vi "Bezier Trajectory.vi"(6 "Overrides":T1 {"Angle Override" step=5.0; "Velocity Override" step=5.0; "Angular Override" step=5.0}, 7 "Drive Type":T4, 8 "Conditions":T7, 9 "All Limits":cluster{"Limits":T2, "Angular Limits":T3} {"Limits"."StoopidFast (fps)" min=0.0; "Limits"."Jerk (fps^3)" min=0.0 step=1.0; "Limits"."Accel (fps^2)" min=0.0; "Limits"."Velocity (fps)" min=0.0; "Angular Limits"."Jerk (deg/s^3)" min=0.0 step=1.0; "Angular Limits"."Accel (deg/s^2)" min=0.0; "Angular Limits"."Velocity (deg/s)" min=0.0}, 10 "sample period (s)":sgl, 11 "WayPoints":T8) -> (0 "Time & Dist":cluster{"Time (s)":dbl, "Distance (ft)":dbl}, 1 "Valid":bool, 2 "Updated Waypoints":cluster{"x":dbl, "y":dbl, "th":dbl}[](array[cluster]), 3 "Trajectory Data":T5)   [LabVIEW 2023]
uses:
  Types/Waypoints.ctl
  Types/Trajectory Data.ctl
  Types/Segment Type.ctl
  Types/Drive Type.ctl
  Types/Limits.ctl
  Types/Angluar Limits.ctl
  Types/Overrides.ctl
panel:
  out "XY Graph":cluster{"X":dbl, "Y":dbl}[](graph)
  in  "dynamic?":bool
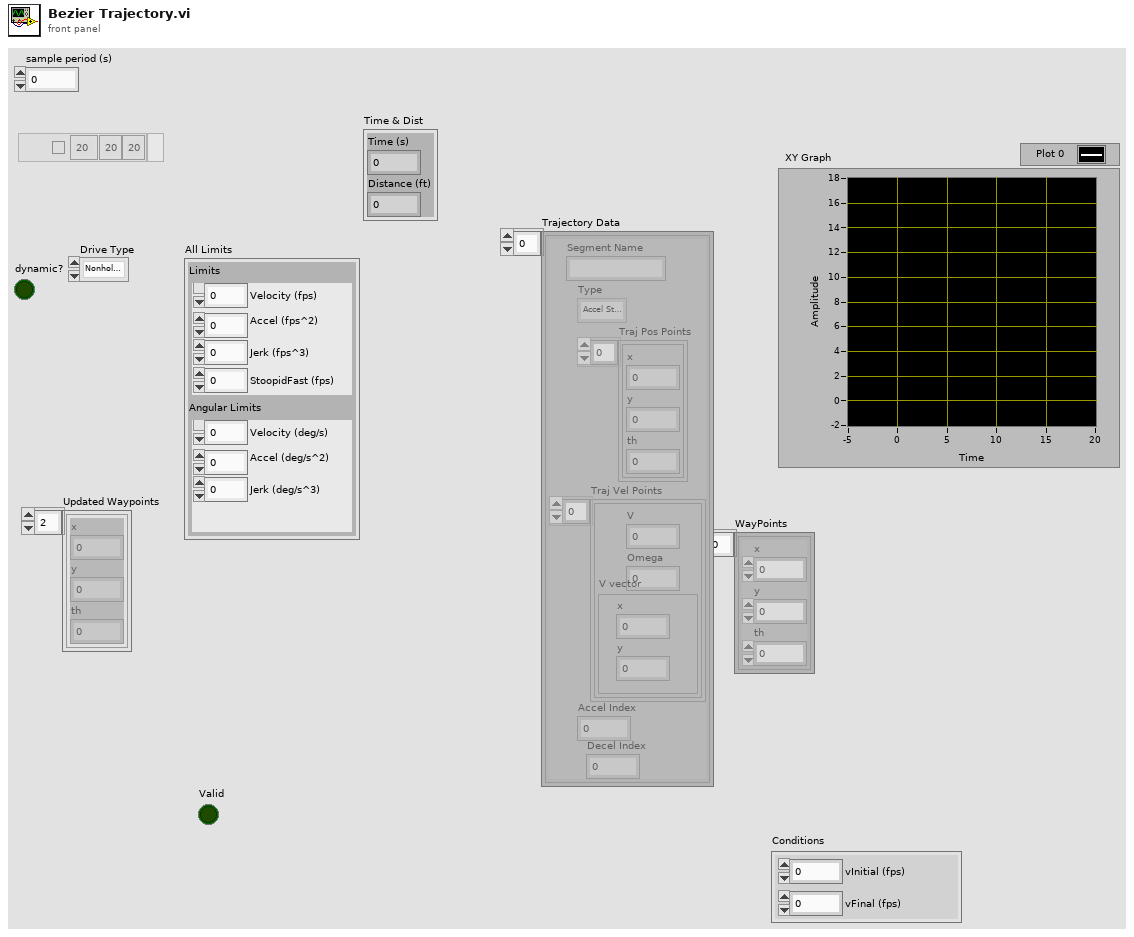
[diagram p1: front panel]
types:
  T1 = typedef "Overrides.ctl" = cluster{"Count":string, "Angular Override":dbl, "Enabled?":bool, "Velocity Override":dbl, "Angle Override":dbl}[]
  T2 = typedef "Limits.ctl" = cluster{"Velocity (fps)":dbl, "Accel (fps^2)":dbl, "Jerk (fps^3)":dbl, "StoopidFast (fps)":dbl}
  T3 = typedef "Angluar Limits.ctl" = cluster{"Velocity (deg/s)":dbl, "Accel (deg/s^2)":dbl, "Jerk (deg/s^3)":dbl}
  T4 = typedef "Drive Type.ctl" = enum16{"Nonholonomic", "Holonomic"}
  T5 = typedef "Trajectory Data.ctl" = cluster{"Segment Name":string, "Type":T6, "Traj Pos Points":cluster{"x":dbl, "y":dbl, "th":dbl}[], "Traj Vel Points":cluster{"V":dbl, "Omega":dbl, "V vector":cluster{"y":dbl, "x":dbl}}[], "Accel Index":i32, "Decel Index":i32}[]
  T6 = typedef "Segment Type.ctl" = enum16{"Accel Straight", "Const Straight", "Blend", "Circle", "Bezier"}
  T7 = cluster{"vInitial (fps)":dbl, "vFinal (fps)":dbl}
  T8 = typedef "Waypoints.ctl" = cluster{"x":sgl, "y":sgl, "th":sgl}[]
  T9 = cluster{"Velocity (fps)":dbl, "Accel (fps^2)":dbl, "Jerk (fps^3)":dbl}
  T10 = typedef "Bezier Curve.ctl" = cluster{"x":sgl, "y":sgl}[]
  T11 = cluster{"Segment Name":string, "Type":T6, "Traj Pos Points":cluster{"x":dbl, "y":dbl, "th":dbl}[], "Traj Vel Points":cluster{"V":dbl, "Omega":dbl, "V vector":cluster{"y":dbl, "x":dbl}}[], "Accel Index":i32, "Decel Index":i32}
  T12 = cluster{"Segment Name":string, "Type":T6, "Traj Pos Points":cluster{"x":dbl, "y":dbl, "th":dbl}[], "Traj Vel Points":cluster{"V":dbl, "Omega":dbl, "V vector":cluster{"y":dbl, "x":dbl}}[], "Accel Index":i32, "Decel Index":i32}[]
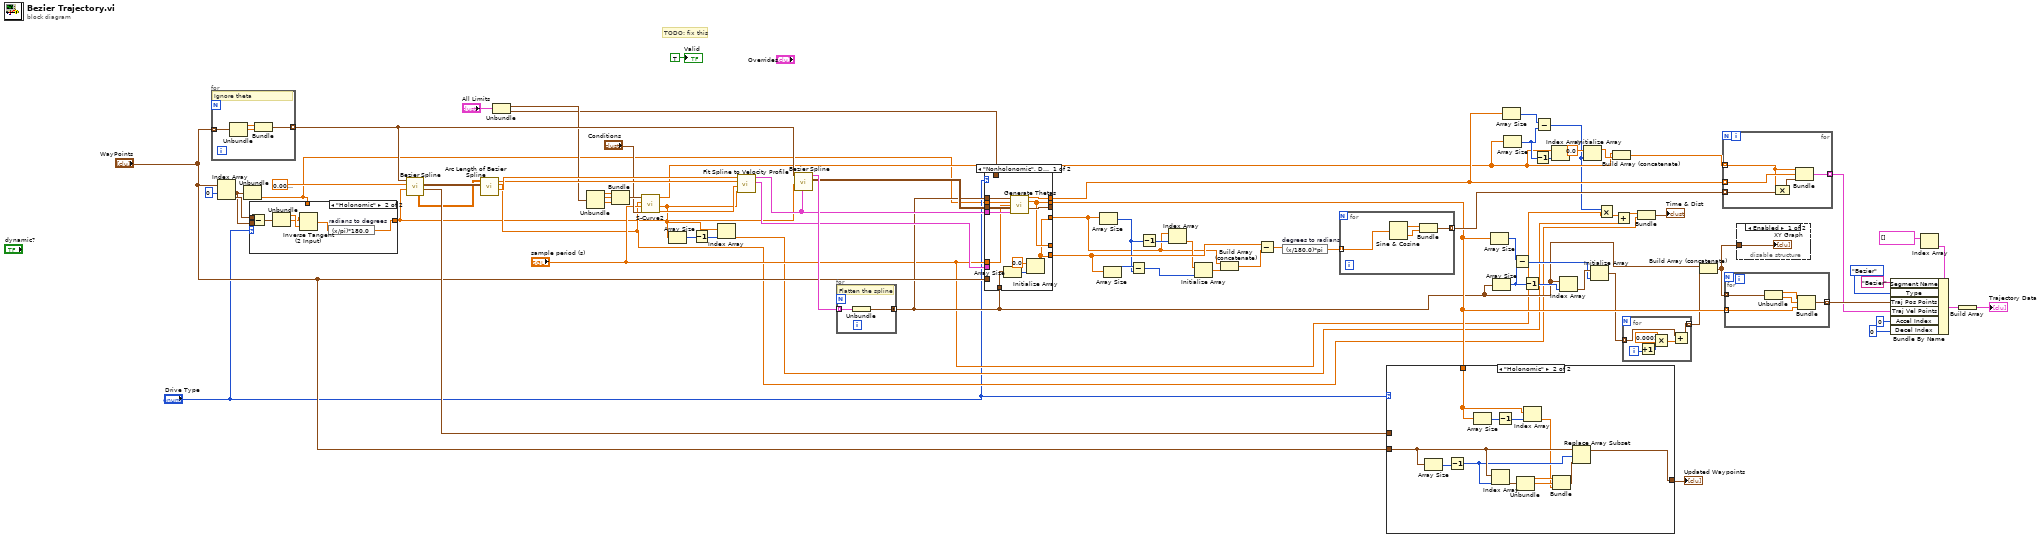
[diagram p0: block diagram]
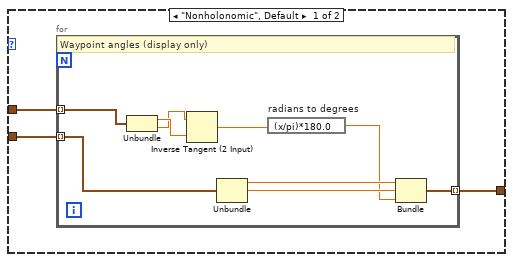
[diagram p4: hidden frame]
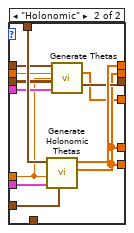
[diagram p5: hidden frame]
diagram:
  # "TODO: fix this"
  n1 = for {
    tunnel: "WayPoints" -> [w83] mode=indexing
    tunnel: [w80] -> w61 mode=indexing
    # "Ignore theta"
    n2 = Unbundle(w83) -> ("x"=w82:sgl, "y"=w81:sgl)  [unwired: 1 out]
    n3 = Bundle("x"=w82, "y"=w81) -> (w80:cluster{"x":sgl, "y":sgl})  [unwired: 1 in]
  }
  n4 = Index Array(array="WayPoints", index #1=0 ("index")) -> (element #1=w4:cluster{"x":sgl, "y":sgl, "th":sgl}, element #2=w5:cluster{"x":sgl, "y":sgl, "th":sgl})  [unwired: 1 in]
  n5 = Unbundle(w4) -> ("th"=w2:sgl)  [unwired: 2 out]
  n6 = case shown="\"Holonomic\"" "Drive Type" {
    tunnel: w5 -> [_ w91]
    tunnel: w4 -> [_ w90]
    tunnel: [w84 w85] -> w1
    tunnel: w2 -> [w84 _]
    frame "Nonholonomic", Default {
    }
    frame "Holonomic" {
      n7 = Subtract(x=w91, y=w90) -> (x-y=w89:cluster{"x":sgl, "y":sgl, "th":sgl})
      n8 = Unbundle(w89) -> ("x"=w88:sgl, "y"=w87:sgl)  [unwired: 1 out]
      n9 = Inverse Tangent (2 Input)(1:w88, 2:w87) -> (0:w86:sgl)
      n10 = expression code="(x/pi)*180.0" "radians to degrees"(w86) -> (w85:sgl)
    }
  }
  n11 = call "Bezier Spline.vi"("starting orientation (deg)"=w1, "percision"=sgl 0.01, "waypts"=w61) -> ("Tangents"=w74:cluster{sgl, sgl}[], "ctrl pts"=w64:cluster{sgl, sgl}[][], "position out"=w58:sgl[][])  [unwired: 4 in, 2 out]
  n12 = call "Arc Length of Bezier Spline.vi"("ctrl pts"=w64, "position"=w58) -> ("t"=w63:sgl[], "l total"=w8:dbl, "l"=w62:dbl[])  [unwired: 6 in, 1 out]
  n13 = Unbundle("All Limits") -> ("Limits"=w51:T2, "Angular Limits"=w50:T3)
  n14 = Unbundle(w51) -> ("Velocity (fps)"=w78:dbl, "Accel (fps^2)"=w77:dbl, "Jerk (fps^3)"=w76:dbl)  [unwired: 1 out]
  n15 = Bundle("Velocity (fps)"=w78, "Accel (fps^2)"=w77, "Jerk (fps^3)"=w76) -> (w75:T9)  [unwired: 1 in]
  n16 = call "S-Curve2.vi"("Conditions"="Conditions", "dt (s)"="sample period (s)", "goal"=w8, "Limits"=w75) -> ("X"=w60:dbl[], "T"=w54:dbl[], "V"=w18:dbl[])  [unwired: 5 in]
  n17 = Array Size(array=w54) -> (size(s)=w73:i32)
  n18 = Decrement(x=w73) -> (x-1=w72:i32)
  n19 = Index Array(array=w54, index=w72) -> (element=w9:dbl)
  n20 = call "Fit Spline to Velocity Profile.vi"("time"=w54, "vel positions"=w60, "s(t)"=w62, "t flat"=w63) -> ("time unflat"=w53:cluster{dbl[]}[], "y unflat"=w55:cluster{dbl[]}[])  [unwired: 6 in]
  n21 = call "Bezier Spline.vi"("positions"=w55, "starting orientation (deg)"=w1, "waypts"=w61) -> ("ctrl pts"=w56:cluster{sgl, sgl}[][], "bezier spline"=w57:cluster{"curve ":T10}[])  [unwired: 4 in, 3 out]
  n22 = for {
    tunnel: w57 -> [w93] mode=indexing
    tunnel: [w92] -> w34 mode=concatenating
    # "Flatten the spline"
    n23 = Unbundle(w93) -> ("curve"=w92:T10)
  }
  n24 = case shown="\"Nonholonomic\", Default" "Drive Type" {
    tunnel: [w105 w117] -> w24
    tunnel: [w99 w108] -> w40
    tunnel: w2 -> [w104 w112]
    tunnel: w34 -> [w103 w113]
    tunnel: w56 -> [w102 w111]
    tunnel: w55 -> [w101 w110]
    tunnel: w53 -> [_ w116]
    tunnel: "sample period (s)" -> [w94 w106]
    tunnel: w50 -> [_ w115]
    tunnel: "WayPoints" -> [_ w114]
    tunnel: [w100 w109] -> _
    tunnel: [w99 w108] -> _
    tunnel: [w95 w108] -> w33
    tunnel: [w95 w107] -> w27
    tunnel: w34 -> [w98 _]
    frame "Nonholonomic", Default {
      n25 = Array Size(array=w98) -> (size(s)=w97:i32)
      n26 = call "Generate Thetas.vi"("spline flat"=w103, "starting angle"=w104, "dt"=w94, "ctrl pts"=w102, "y unflat"=w101) -> ("omega"=w105:sgl[], "theta"=w99:sgl[], "Tangent Vector"=w100:cluster{"x out":dbl, "y out":dbl}[])  [unwired: 8 in]
      n27 = Initialize Array(0.0 ("element"), w97) -> (w95:dbl[])
    }
    frame "Holonomic" {
      n28 = call "Generate Holonomic Thetas.vi"("WayPoints"=w114, "time unflat"=w116, "dt"=w106, "Angular Limits"=w115) -> ("X"=w108:dbl[], "V"=w117:dbl[])  [unwired: 6 in]
      n29 = call "Generate Thetas.vi"("spline flat"=w113, "starting angle"=w112, "dt"=w106, "ctrl pts"=w111, "y unflat"=w110) -> ("theta"=w107:sgl[], "Tangent Vector"=w109:cluster{"x out":dbl, "y out":dbl}[])  [unwired: 8 in, 1 out]
    }
  }
  n30 = Array Size(array=w27) -> (size(s)=w30:i32)
  n31 = Array Size(array=w33) -> (size(s)=w32:i32)
  n32 = Subtract(x=w32, y=w30) -> (x-y=w31:i32)
  n33 = Decrement(x=w30) -> (x-1=w29:i32)
  n34 = Index Array(array=w27, index=w29) -> (element=w28:dbl)
  n35 = Initialize Array(w28, w31) -> (w26:dbl[])
  n36 = Build Array (concatenate)(w27, w26) -> (w25:dbl[])
  n37 = Subtract(x=w33, y=w25) -> (x-y=w41:dbl[])
  n38 = expression code="(x/180.0)*pi" "degrees to radians"(w41) -> (w42:dbl[])
  n39 = for {
    tunnel: w42 -> [w119] mode=indexing
    tunnel: [w121] -> w43 mode=indexing
    n40 = Sine & Cosine(0:w119) -> (1:w120:dbl, 2:w118:dbl)
    n41 = Bundle(w120, w118) -> (w121:cluster{dbl, dbl})  [unwired: 1 in]
  }
  n42 = case shown="\"Holonomic\"" "Drive Type" {
    tunnel: w74 -> [w124 _]
    tunnel: "WayPoints" -> [w123 w141]
    tunnel: [w122 w134] -> w49
    tunnel: w40 -> [_ w143]
    frame "Nonholonomic", Default {
      n43 = for {
        tunnel: w123 -> [w133] mode=indexing
        tunnel: w124 -> [w125] mode=indexing
        tunnel: [w130] -> w122 mode=indexing
        # "Waypoint angles (display only)"
        n44 = Unbundle(w125) -> (w128:sgl, w127:sgl)
        n45 = Inverse Tangent (2 Input)(1:w128, 2:w127) -> (0:w126:sgl)
        n46 = Unbundle(w133) -> ("x"=w132:sgl, "y"=w131:sgl)  [unwired: 1 out]
        n47 = expression code="(x/pi)*180.0" "radians to degrees"(w126) -> (w129:sgl)
        n48 = Bundle("x"=w132, "y"=w131, w129) -> (w130:cluster{"x":sgl, "y":sgl, sgl})  [unwired: 1 in]
      }
    }
    frame "Holonomic" {
      n49 = Array Size(array=w141) -> (size(s)=w142:i32)
      n50 = Decrement(x=w142) -> (x-1=w140:i32)
      n51 = Array Size(array=w143) -> (size(s)=w145:i32)
      n52 = Index Array(array=w141, index=w140) -> (element=w139:cluster{"x":sgl, "y":sgl, "th":sgl})
      n53 = Decrement(x=w145) -> (x-1=w144:i32)
      n54 = Unbundle(w139) -> ("x"=w138:sgl, "y"=w137:sgl)  [unwired: 1 out]
      n55 = Index Array(array=w143, index=w144) -> (element=w136:dbl)
      n56 = Bundle("x"=w138, "y"=w137, w136) -> (w135:cluster{"x":sgl, "y":sgl, dbl})  [unwired: 1 in]
      n57 = Replace Array Subset(array=w141, new element=w135, index=w140) -> (w134:T8)
    }
  }
  "Updated Waypoints" <- w49
  n58 = Array Size(array=w40) -> (size(s)=w39:i32)
  n59 = Array Size(array=w34) -> (size(s)=w38:i32)
  n60 = Array Size(array=w24) -> (size(s)=w23:i32)
  n61 = Array Size(array=w18) -> (size(s)=w22:i32)
  n62 = Subtract(x=w39, y=w38) -> (x-y=w35:i32)
  n63 = Decrement(x=w38) -> (x-1=w37:i32)
  n64 = Decrement(x=w22) -> (x-1=w21:i32)
  n65 = Subtract(x=w23, y=w22) -> (x-y=w14:i32)
  n66 = Index Array(array=w18, index=w21) -> ()  [unwired: 1 out]
  n67 = Index Array(array=w34, index=w37) -> (element=w36:cluster{"x":sgl, "y":sgl})
  n68 = Initialize Array(0.0 ("element"), w14) -> (w20:dbl[])
  n69 = Initialize Array(w36, w35) -> (w16:cluster{"x":sgl, "y":sgl}[])
  n70 = Multiply(x=w14, y="sample period (s)") -> (x*y=w13:sgl)
  n71 = Build Array (concatenate)(w18, w20) -> (w17:dbl[])
  n72 = Add(x=w13, y=w9) -> (x+y=w12:dbl)
  n73 = for {
    tunnel: w16 -> [w147] mode=indexing
    tunnel: [w146] -> w15 mode=indexing
    i -> [w150]
    n74 = Increment(x=w150) -> (x+1=w149:i32)
    n75 = Multiply(x=0.0001, y=w149) -> (x*y=w148:dbl)
    n76 = Add(x=w147, y=w148) -> (x+y=w146:cluster{"x":dbl, "y":dbl})
  }
  n77 = Bundle(w12, "l total"=w8) -> (→"Time & Dist":cluster{dbl, "l total":dbl})  [unwired: 1 in]
  n78 = Build Array (concatenate)(w34, w15) -> (w7:cluster{"x":dbl, "y":dbl}[])
  n79 = for {
    tunnel: w24 -> [w156] mode=indexing
    tunnel: w17 -> [w152] mode=indexing
    tunnel: [w155] -> w67 mode=indexing
    tunnel: w43 -> [w153] mode=indexing
    n80 = Compound Arithmetic op=MULTIPLY(w152, w153) -> (w154:cluster{dbl, dbl})
    n81 = Bundle("element"=w152, w156, w154) -> (w155:cluster{"element":dbl, dbl, cluster{dbl, dbl}})  [unwired: 1 in]
  }
  n82 = for {
    tunnel: w7 -> [w161] mode=indexing
    tunnel: [w158] -> w68 mode=indexing
    tunnel: w40 -> [w157] mode=indexing
    n83 = Unbundle(w161) -> ("x"=w160:dbl, "y"=w159:dbl)
    n84 = Bundle("x"=w160, "y"=w159, w157) -> (w158:cluster{"x":dbl, "y":dbl, dbl})  [unwired: 1 in]
  }
  n85 = disable-structure shown="Enabled" {
    disable-tunnel: w7 -> [w162 _]
    frame Enabled {
      "XY Graph" <- w162
    }
    frame Disabled {
    }
  }
  n86 = Index Array(array=T5 [] ("Trajectory Data")) -> (element=w44:T11)  [unwired: 1 in]
  n87 = Bundle By Name(cluster=w44, "Segment Name"="Bezier", "Type"=Segment_Type."Bezier", "Traj Pos Points"=w68, "Traj Vel Points"=w67, "Accel Index"=0, "Decel Index"=0) -> (w6:T11)
  n88 = Build Array(w6) -> (→"Trajectory Data":T12)
  "Valid" <- TRUE ("Valid")
